vi "Phasor Compute Calibrated SDV [(m, phi) cal].vi"(8 "error in":errorcluster, 9 "Calibration Phasor":T1, 11 "Raw Phasor":T2) -> (0 "error out":errorcluster, 3 "Calibrated Phasor SDV (g, s)":T2)   [LabVIEW 2021, in "Phasor.lvlib"]
uses:
  Phasor.lvlib
  Phasor (g, s).ctl
  Calibration Phasor (m, phi).ctl
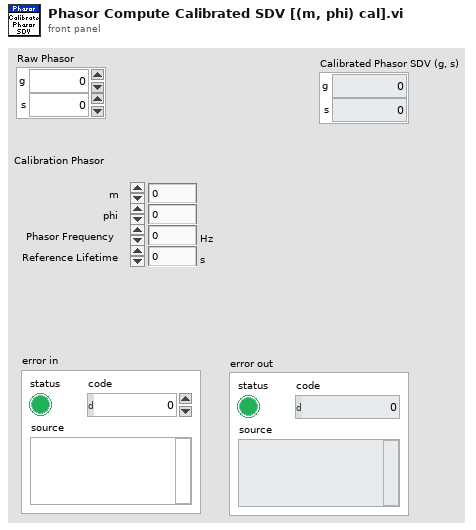
[diagram p1: front panel]
types:
  T1 = typedef "Phasor.lvlib/Calibration Phasor (m, phi).ctl" = cluster{"m":dbl, "phi":dbl, "Phasor Frequency":dbl[unit], "Reference Lifetime":dbl[unit]}
  T2 = typedef "Phasor.lvlib/Phasor (g, s).ctl" = cluster{"g":dbl, "s":dbl}
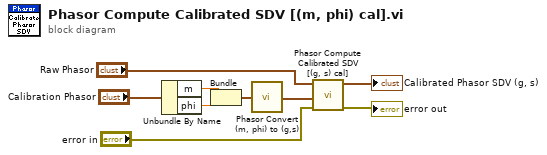
[diagram p0: block diagram]
diagram:
  n1 = Unbundle By Name("Calibration Phasor") -> ("m"=w3:dbl, "phi"=w4:dbl)
  n2 = Bundle("m"=w3, "phi"=w4) -> (w5:cluster{"m":dbl, "phi":dbl})  [unwired: 1 in]
  n3 = call "Phasor Convert (m, phi) to (g,s).vi"("Phasor (m, phi)"=w5) -> ("Phasor (g, s)"=w2:T2)  [unwired: 8 in]
  n4 = call "Phasor Compute Calibrated SDV [(g, s) cal].vi"("Error In"="error in", "Phasor Calibration (g,s)"=w2, "Raw Phasor SDV (g, s)"="Raw Phasor") -> ("Error Out"=→"error out":errorcluster, "Calibrated Phasor SDV (g, s)"=→"Calibrated Phasor SDV (g, s)":T2)  [unwired: 7 in]
